vi "Shared_DCPower_Configure.vi"(7 "DCPower Parameters":T1[](array[typedef]) {"Source Delay" format="%.6p"; "Sense" items=["Local"=1008, "Remote"=1009]; "Aperture_time" format="%.6p"; "Current_range" format="%.6p"; "Current" format="%.6p"; "Voltage_range" format="%.6p"; "Voltage" format="%.6p"}, 8 "trigger out?":bool, 9 "output terminal":tag[](array[tag]), 10 "Pins":tag[](array[tag]), 11 "Semiconductor Module Context":T2) -> (0 "error Out":errorcluster)   [LabVIEW 2020, in "Shared.lvlib"]
doc: "Configure the System Power Supply for Relay control"
uses:
  Shared.lvlib
  <vilib>/NI_TestStand_SemiconductorModule/NI_TestStand_Semiconductor_Module.lvlibp/PinMap/General/SemiconductorModuleContext.ctl
  ResourceHandling/TypeDefs/RH_DCPower_Parameters.ctl
  <vilib>/NI_TestStand_SemiconductorModule/NI_TestStand_Semiconductor_Module.lvlibp/PinMap/DC Power/PinsToNIDCPowerSessions.vi
  <vilib>/NI_TestStand_SemiconductorModule/NI_TestStand_Semiconductor_Module.lvlibp
  ResourceHandling/ResourceHandling.lvlib
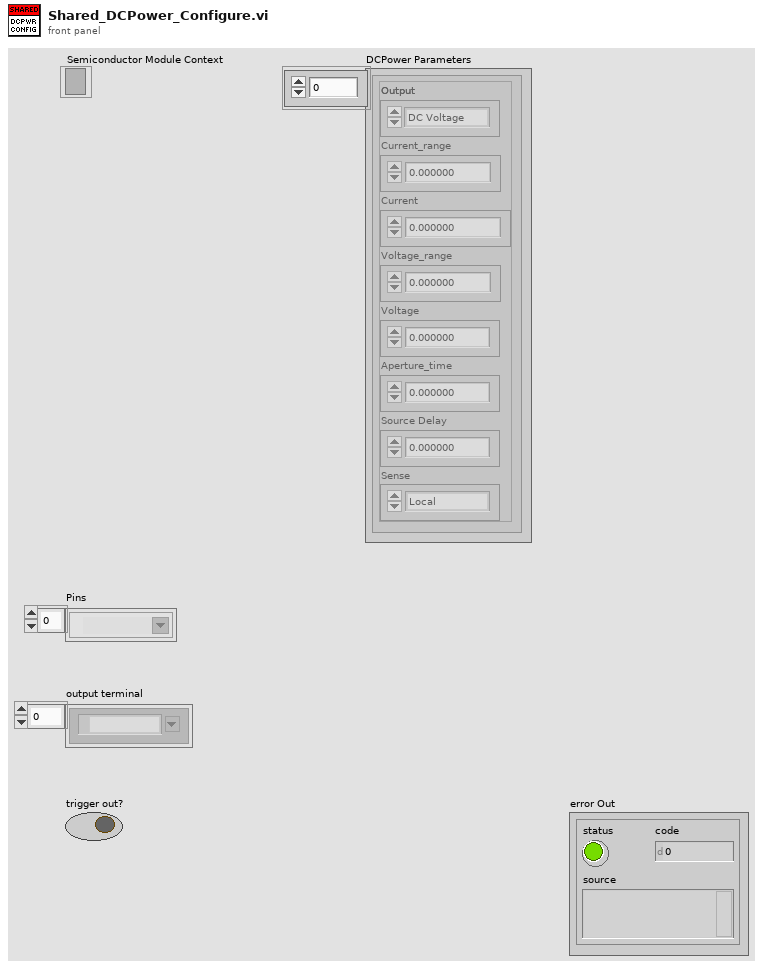
[diagram p1: front panel]
types:
  T1 = typedef "ResourceHandling.lvlib/RH_DCPower_Parameters.ctl" = cluster{"Output":enum16{"DC Voltage", "DC Current"}, "Current_range":dbl, "Current":dbl, "Voltage_range":dbl, "Voltage":dbl, "Aperture_time":dbl, "Source Delay":dbl, "Sense":i32}
  T2 = typedef "NI_TestStand_Semiconductor_Module.lvlibp/SemiconductorModuleContext.ctl" = refnum<k7>
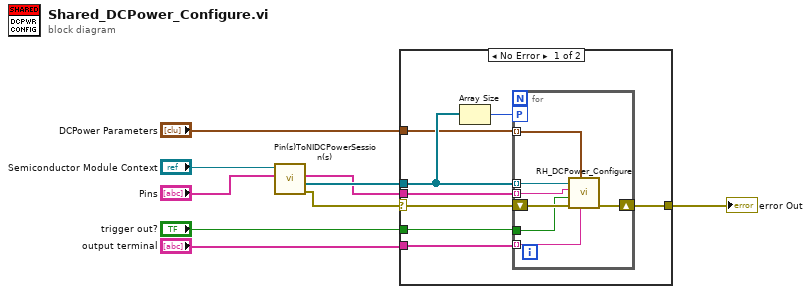
[diagram p0: block diagram]
diagram:
  n1 = call-poly <vilib>:"Pin(s)ToNIDCPowerSession(s).vi"("Pins"="Pins", "Semiconductor Module Context"="Semiconductor Module Context") -> ("error out"=w8:errorcluster, "Instrument Sessions"=w7:refnum<k15>[], "Channel Strings"=w6:string[])  [unwired: 5 in, 2 out]
  n2 = case shown="No Error" w8 {
    selector: w8 -> [w13 w25]
    tunnel: w7 -> [w16 _]
    tunnel: w6 -> [w15 _]
    tunnel: [w14 w25] -> w5
    tunnel: "DCPower Parameters" -> [w12 _]
    tunnel: "trigger out?" -> [w11 _]
    tunnel: "output terminal" -> [w10 _]
    frame No Error {
      n3 = Array Size(array=w16) -> (size(s)=w17:i32)
      n4 = for {
        tunnel: w16 -> [w24] mode=indexing
        workers-P: w17 -> [_]
        tunnel: w15 -> [w23] mode=indexing
        shift-right: [w22] -> w14
        shift-left: w13 -> [w21]
        tunnel: w12 -> [w20] mode=indexing
        tunnel: w11 -> [w19]
        tunnel: w10 -> [w18] mode=indexing
        n5 = call "RH_DCPower_Configure.vi"("output terminal"=w18, "DCPower_Parameters"=w20, "error in (no error)"=w21, "trigger out?"=w19, "channel name"=w23, "DCPower Session In"=w24) -> ("error out"=w22:errorcluster)  [unwired: 4 in, 1 out]
      }
    }
    frame Error {
    }
  }
  "error Out" <- w5
